vi "VerifyArguments.vi"(8 "error in (no error)":errorcluster, 11 "VIPMInstallPackageFile in":refnum<class "VIPMInstallPackageFile.lvclass">) -> (0 "error out":errorcluster, 3 "VIPMInstallPackageFile out":refnum<class "VIPMInstallPackageFile.lvclass">)   [LabVIEW 2014, in "VIPMInstallPackageFile.lvclass"]
uses:
  <nishared>/LabVIEW CLI/Operations/VIPMInstallPackageFile/VIPMInstallPackageFile.lvclass
  <nishared>/LabVIEW CLI/Operations/VIPMInstallPackageFile/VIPMInstallPackageFile.lvclass/VIPMInstallPackageFile.ctl
  <nishared>/LabVIEW CLI/Operations/Utilities/OperationErrorType.ctl
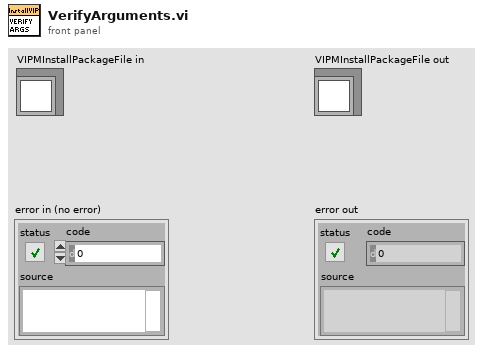
[diagram p1: front panel]
types:
  T1 = typedef "OperationErrorType.ctl" = enum16{"RequiredArgumentMissing", "UnknownArguments", "LoggerSetMultipleTimes", "OperationBrokenError"}
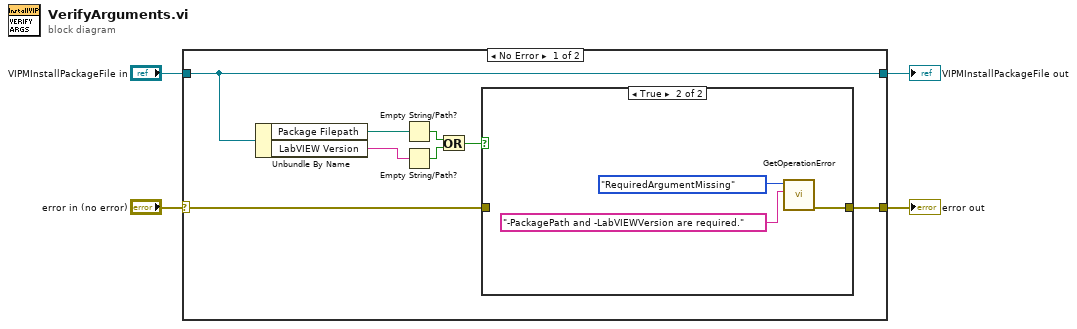
[diagram p0: block diagram]
diagram:
  n1 = case shown="No Error" "error in (no error)" {
    selector: "error in (no error)" -> [w9 w18]
    tunnel: [w10 w18] -> w3
    tunnel: "VIPMInstallPackageFile in" -> [w12 w17]
    tunnel: [w12 w17] -> w1
    frame No Error {
      n2 = Unbundle By Name(w12) -> ("Package Filepath"=w11:path, "LabVIEW Version"=w8:string)
      n3 = Empty String/Path?(string/path=w11) -> (empty?=w7:bool)
      n4 = Empty String/Path?(string/path=w8) -> (empty?=w6:bool)
      n5 = Or(x=w7, y=w6) -> (x .or. y?=w5:bool)
      n6 = case shown="True" w5 {
        tunnel: [w13 w14] -> w10
        tunnel: w9 -> [w13 _]
        frame False {
        }
        frame True {
          n7 = call <nishared>:"GetOperationError.vi"("Additional Information"="-PackagePath and -LabVIEWVersion are required.", "Operation Error Type"=OperationErrorType."RequiredArgumentMissing") -> ("error out"=w14:errorcluster)  [unwired: 9 in]
        }
      }
    }
    frame Error {
    }
  }
  "error out" <- w3
  "VIPMInstallPackageFile out" <- w1
